vi "power analyzer.vi"() -> ()   [LabVIEW 2011]
uses:
  <instrlib>/Voltech PM1000+/Voltech PM1000+.lvlib
  <vilib>/Utility/file.llb/Write To Spreadsheet File (string).vi
panel:
  out "Array":string[](array[string])
  out "Measurement Results":string[][](array[string])
  in  "Set Start Time (s)":dbl
  in  "Time Target (s)":dbl=8.0
  out "stripped path":path
  out "error out":errorcluster
  in  "VISA resource name 2":refnum<visa-resource-name>
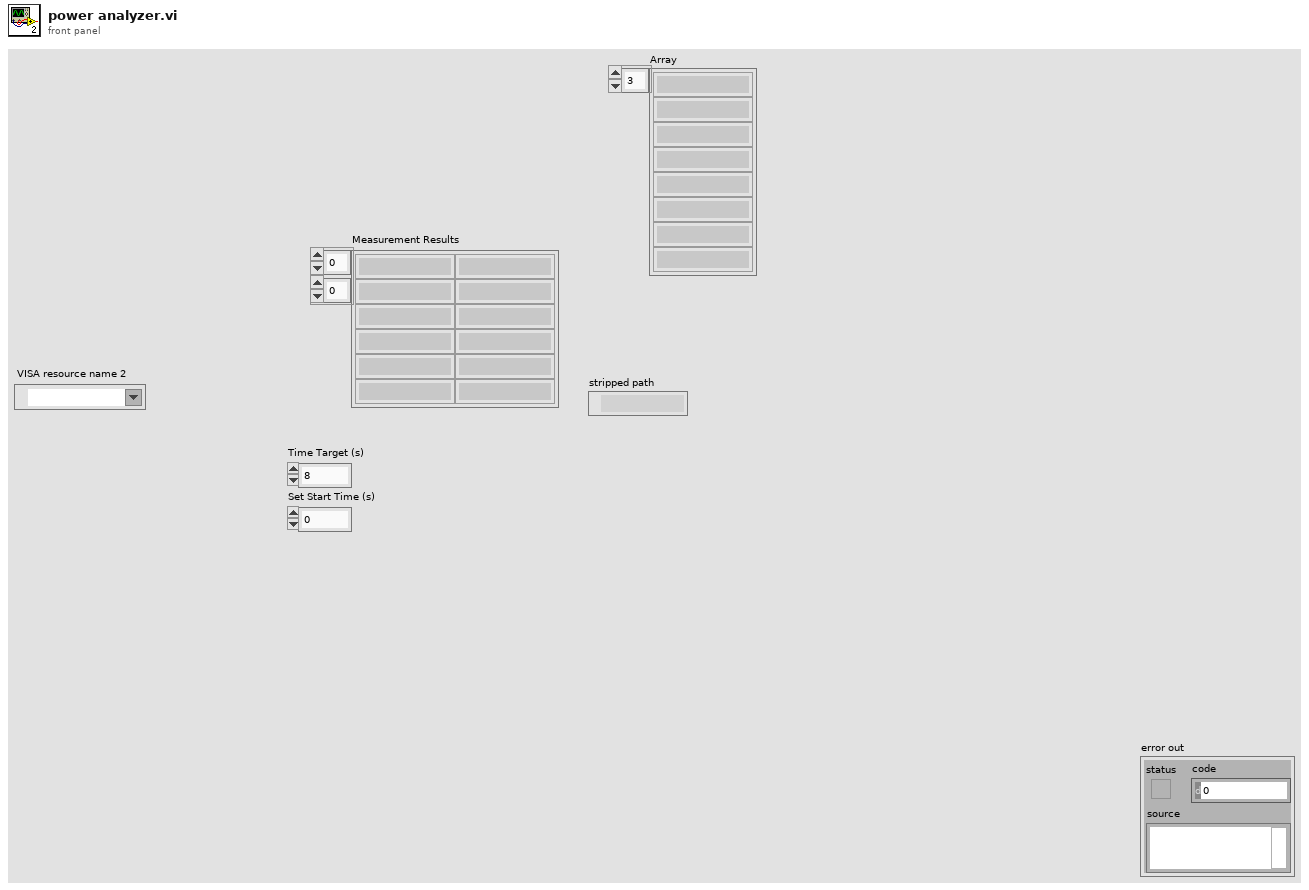
[diagram p1: front panel]
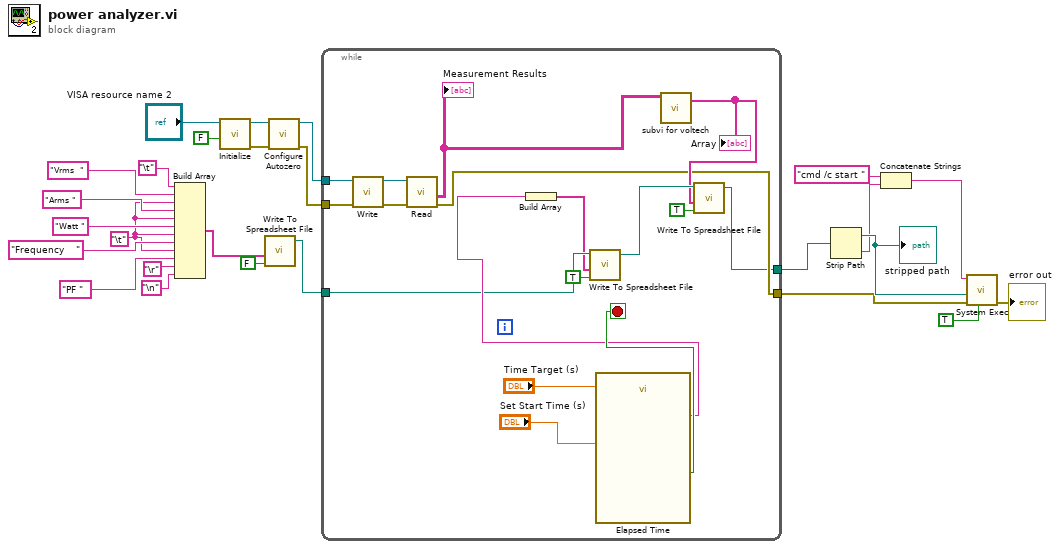
[diagram p0: block diagram]
diagram:
  w22 = "\t"
  n1 = Build Array("\t", "Vrms  " ("string"), w22, "Arms " ("string"), w22, "Watt " ("string"), w22, "Frequency    " ("string"), w22, "PF " ("string"), "\r", "\n") -> (w6:string[])
  n2 = call <instrlib>:"Initialize.vi"("Reset (True)"=FALSE, "VISA resource name"="VISA resource name 2") -> ("error out"=w17:errorcluster, "VISA resource name out"=w16:refnum<visa-resource-name>)  [unwired: 8 in]
  n3 = call-poly <vilib>:"Write To Spreadsheet File.vi"("append to file? (new file:F)"=FALSE, "1D data"=w6) -> ("new file path (Not A Path if cancelled)"=w4:path)  [unwired: 6 in]
  n4 = call <instrlib>:"Configure Autozero.vi"("error in (no error)"=w17, "VISA resource name"=w16) -> ("error out"=w13:errorcluster, "VISA resource name out"=w14:refnum<visa-resource-name>)  [unwired: 8 in]
  n5 = while {
    tunnel: w14 -> [w41]
    tunnel: w13 -> [w40]
    tunnel: w4 -> [w35]
    tunnel: [w28] -> w3
    tunnel: [w27] -> w2
    stop <- w37 stop-if-true
    n6 = call <instrlib>:"Write.vi"("error in (no error)"=w40, "VISA resource name"=w41) -> ("error out"=w42:errorcluster, "VISA resource name out"=w43:refnum<visa-resource-name>)  [unwired: 8 in]
    n7 = call <instrlib>:"Read.vi"("error in (no error)"=w42, "VISA resource name"=w43) -> ("error out"=w28:errorcluster, "Measurement Results"=w31:string[][])  [unwired: 7 in, 1 out]
    "Measurement Results" <- w31
    n8 = call "Elapsed Time"("Time Target (s)"="Time Target (s)", "Set Start Time (s)"="Set Start Time (s)") -> ("Time has Elapsed"=w37:bool, "Elapsed Time Text"=w36:string)  [unwired: 10 in, 6 out]
    n9 = Build Array(w36) -> (w33:string[])
    n10 = call-poly <vilib>:"Write To Spreadsheet File.vi"("append to file? (new file:F)"=TRUE, "1D data"=w33, "file path (dialog if empty)"=w35) -> ("new file path (Not A Path if cancelled)"=w32:path)  [unwired: 5 in]
    n11 = call "subvi for voltech.vi"("Measurement Results 2"=w31) -> ("Array"=w30:string[])  [unwired: 5 in]
    "Array" <- w30
    n12 = call-poly <vilib>:"Write To Spreadsheet File.vi"("append to file? (new file:F)"=TRUE, "1D data"=w30, "file path (dialog if empty)"=w32) -> ("new file path (Not A Path if cancelled)"=w27:path)  [unwired: 5 in]
  }
  n13 = Strip Path(path=w2) -> (stripped path=w11:path, name=w10:string)
  "stripped path" <- w11
  n14 = Concatenate Strings("cmd /c start " ("string"), w10) -> (w9:string)
  n15 = call <vilib>:"System Exec.vi"("run minimized? (F)"=TRUE, "error in (no error)"=w3, "working directory"=w11, "command line"=w9) -> ("error out"=→"error out":errorcluster)  [unwired: 4 in, 3 out]
